vi "Biometry Configuration.vi"(8 "error in (no error)":errorcluster caption="错误输入（无错误）") -> (0 "error out":errorcluster caption="错误输出", 3 "Biometry Configuration":T1)   [LabVIEW 2015, in "Boimetry Processing.lvlib"]
doc: "通过读取XML文件，设置眼轴信号测量计算的参数。\n输出Biometry计算的设置参数。"
uses:
  Boimetry Processing.lvlib
  Controls/Biometry Configuration.ctl
  Utility VIs/Utility VIs.lvlib
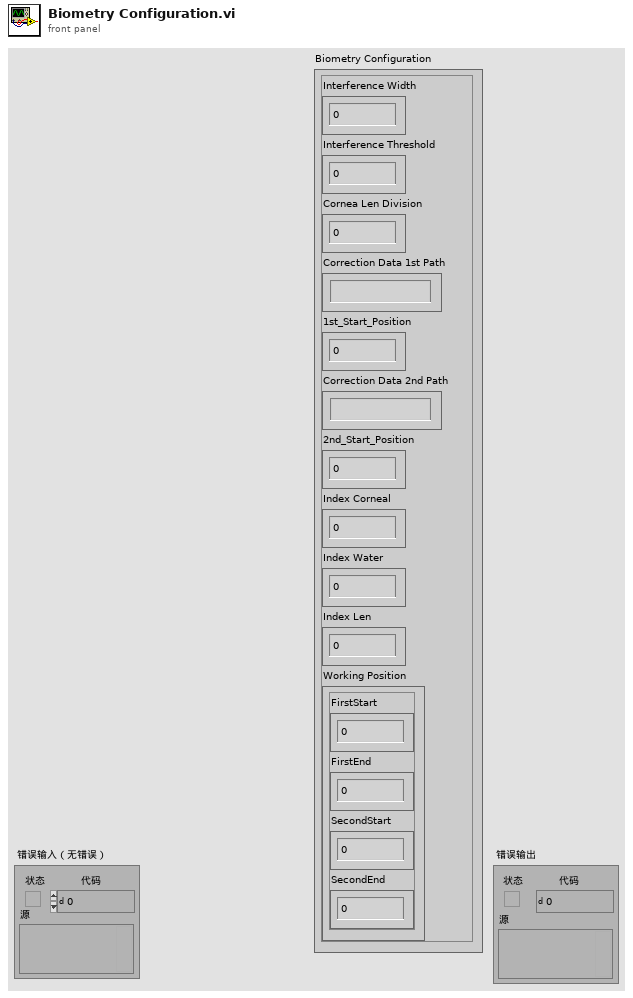
[diagram p1: front panel]
types:
  T1 = typedef "Boimetry Processing.lvlib/Biometry Configuration.ctl" = cluster{"Interference Width":i32, "Interference Threshold":dbl, "Cornea Len Division":i32, "Correction Data 1st Path":string, "1st_Start_Position":dbl, "Correction Data 2nd Path":string, "2nd_Start_Position":dbl, "Index Corneal":dbl, "Index Water":dbl, "Index Len":dbl, "Working Position":cluster{"FirstStart":i32, "FirstEnd":i32, "SecondStart":i32, "SecondEnd":i32}}
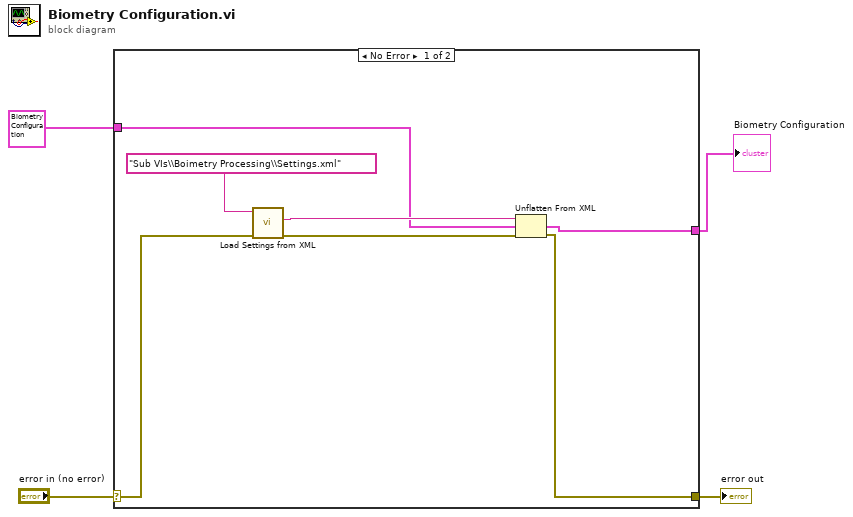
[diagram p0: block diagram]
diagram:
  n1 = case shown="No Error" "error in (no error)" {
    selector: "error in (no error)" -> [w7 w12]
    tunnel: [w6 w12] -> w3
    tunnel: T1 {"Interference Width"=0, "Interference Threshold"=0.0, "Cornea Len Division"=0, "Correction Data 1st Path"="", "1st_Start_Position"=0.0, "Correction Data 2nd Path"="", "2nd_Start_Position"=0.0, "Index Corneal"=0.0, "Index Water"=0.0, "Index Len"=0.0, "Working Position"={"FirstStart"=0, "FirstEnd"=0, "SecondStart"=0, "SecondEnd"=0}} ("Biometry Configuration") -> [w9 _]
    tunnel: [w5 _] -> w2
    frame No Error {
      n2 = call "Load Settings from XML.vi"("error in (no error)"=w7, "名称或相对路径"="Sub VIs\\Boimetry Processing\\Settings.xml") -> ("error out"=w8:errorcluster, "XML Elements"=w10:string)  [unwired: 8 in]
      n3 = Unflatten From XML(xml string=w10, type=w9, error in (no error)=w8) -> (value=w5:T1, error out=w6:errorcluster)
    }
    frame Error {
    }
  }
  "error out" <- w3
  "Biometry Configuration" <- w2
